vi "PH_PowerUnit_BaseClass.PC Timeout SM.vi"(0 "VI in":refnum<vi>, 2 "Timeout SM":T1, 5 "error in (no error)":errorcluster) -> (14 "VI out":refnum<vi>, 19 "error out":errorcluster)   [LabVIEW 2014, in "PH_PowerUnit_BaseClass.lvlib"]
uses:
  PH_PowerUnit_BaseClass.lvlib
  PH_PowerUnit_BaseClass.SM States.ctl
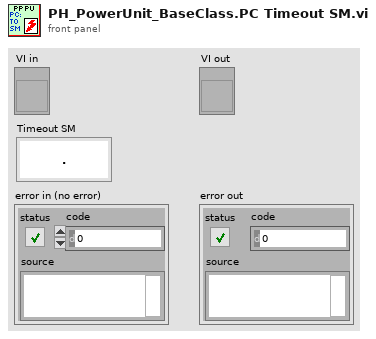
[diagram p1: front panel]
types:
  T1 = typedef "PH_PowerUnit_BaseClass.lvlib/PH_PowerUnit_BaseClass.SM States.ctl" = enum16{".", "Stand by", "Switch PU on", "Configure", "Set Default Voltage", "Set STANDBY", "Set READY", "Wait for Shot Cmd", "Open Dump Rods", "Open Ross Relais", "Close Ross Relais", "Switch PSU on", "Switch PSU off", "Charge", "Switch GD Channel on", "Close Dump Rods", "Rods-TO", "RR-TO", "PSU-TO", "Trigger-TO"}
  T2 = typedef "PH_PowerUnit_BaseClass.lvlib/PH_PowerUnit_BaseClass.i attribute.ctl" = cluster{"Constructor finished":bool, "PU":cluster{"In use":bool, "Service ID in use":i32, "GUI Ref":refnum<vi>}, "Enabling":cluster{"State":T3, "GUI Ref":refnum<vi>}, "Timing":cluster{"Last Shot":dbl, "Time between Shots [Sec]":dbl, "Waiting Time over?":bool, "Service ID Waiting Time":i32, "GUI Ref":refnum<vi>, "Instance":cluster{"Status":T4, "linked?":bool, "GUI Ref":refnum<vi>}}, "Sequencer":cluster{"SM State":string, "GUI Ref":refnum<vi>, "linked":bool}, "Subscribed Trendmssgs":cluster{"Tagname":string, "Status":T4, "linked?":bool, "Shot Condition":T4, "GUI Ref":refnum<vi>}[], "PP PU":T5, "Default Voltage (V)":dbl, "GUI Refs":T6, "PSDB data":cluster{"Shot Voltage [V]":dbl, "State TO SM":T1, "Write 2 early":bool}, "State TO SM":T1}
  T3 = typedef "PH_SystemInformation.lvlib/PH_SystemInformationEnabling State.ctl" = i32
  T4 = typedef "PH_StatusHandler.lvlib/PH_StatusHandler.Status.ctl" = i16
  T5 = typedef "PH_PP_Common.lvlib/PH_PP_Common.PUs.ctl" = enum16{"no Info", "PA-19mm-1", "PA-19mm-2", "PA-45mm-PILC", "PA-45mm-MAIN", "MA-PU-1", "MA-PU-2", "MA-PU-3", "MA-PU-4", "MA-PU-5", "MA-PU-6", "MA-FR", "MA-PILC", "PA-45mm-DP"}
  T6 = typedef "PH_PowerUnit_BaseClass.lvlib/PH_PowerUnit_BaseClass.GUI Refs.ctl" = cluster{"Delete Inst":refnum<vi>, "State TO SM":refnum<vi>, "State SM":refnum<vi>, "Fire":refnum<vi>}
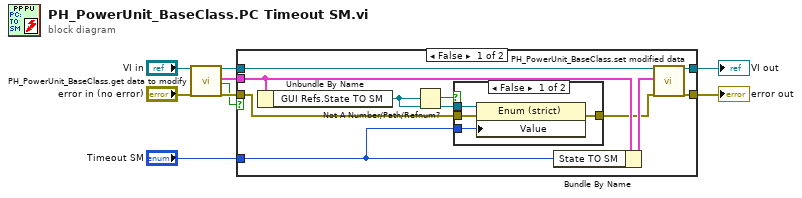
[diagram p0: block diagram]
diagram:
  n1 = call "PH_PowerUnit_BaseClass.get data to modify.vi"("i ref in"="VI in", "error in (no error)"="error in (no error)") -> ("i ref out"=w2:refnum<vi>, "i attribute"=w3:T2, "timed out"=w1:bool, "error out"=w4:errorcluster)  [unwired: 14 in]
  n2 = case shown="False" w1 {
    tunnel: w2 -> [w19 w26]
    tunnel: [w18 w26] -> w6
    tunnel: w4 -> [w12 w25]
    tunnel: [w17 w25] -> w7
    tunnel: w3 -> [w15 _]
    tunnel: "Timeout SM" -> [w13 _]
    frame False {
      n3 = Unbundle By Name(w15) -> ("GUI Refs.State TO SM"=w10:refnum<vi>)
      n4 = Not A Number/Path/Refnum?(number/path/refnum=w10) -> (NaN/Path/Refnum?=w11:bool)
      n5 = case shown="False" w11 {
        tunnel: [w23 w24] -> w14
        tunnel: w10 -> [w22 _]
        tunnel: w13 -> [w21 _]
        tunnel: w12 -> [w20 w24]
        frame False {
          n6 = property class="Enum (strict)"(reference=w22, error in=w20, "Value"=w21) -> (error out=w23:errorcluster)  [unwired: 1 out]
        }
        frame True {
        }
      }
      n7 = Bundle By Name(cluster=w15, "State TO SM"=w13) -> (w16:T2)
      n8 = call "PH_PowerUnit_BaseClass.set modified data.vi"("i ref in"=w19, "i attribute"=w16, "error in (no error)"=w14) -> ("i ref out"=w18:refnum<vi>, "error out"=w17:errorcluster)  [unwired: 15 in]
    }
    frame True {
    }
  }
  "error out" <- w7
  "VI out" <- w6
